vi "Destroy.vi"(8 "error in (no error)":errorcluster, 9 "force destroy? (F)":bool, 11 "State in":refnum<class "State.lvclass">) -> (0 "error out":errorcluster)   [LabVIEW 2017, in "Promise Future.lvlib" / "State.lvclass"]
uses:
  State.lvclass
  State.lvclass/State.ctl
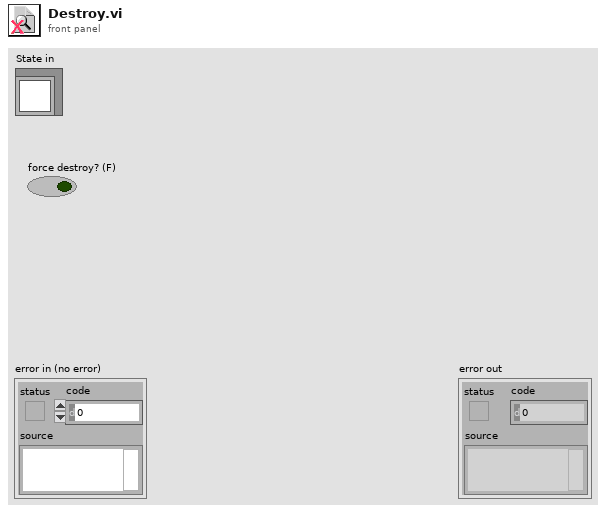
[diagram p1: front panel]
types:
  T1 = typedef "Semaphore RefNum" = refnum<k1>
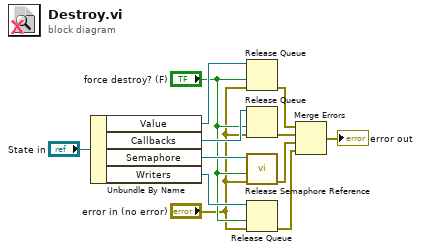
[diagram p0: block diagram]
diagram:
  n1 = Unbundle By Name("State in") -> ("Value"=w11:refnum<queue>, "Callbacks"=w9:refnum<queue>, "Semaphore"=w8:T1, "Writers"=w10:refnum<queue>)
  n2 = Release Queue(queue=w11, force destroy? (F)="force destroy? (F)", error in (no error)="error in (no error)") -> (error out=w6:errorcluster)  [unwired: 2 out]
  n3 = Release Queue(queue=w9, force destroy? (F)="force destroy? (F)", error in (no error)="error in (no error)") -> (error out=w5:errorcluster)  [unwired: 2 out]
  n4 = call <vilib>:"Release Semaphore Reference.vi"("error in (no error)"="error in (no error)", "force destroy? (F)"="force destroy? (F)", "semaphore"=w8) -> ("error out"=w4:errorcluster)  [unwired: 7 in, 1 out]
  n5 = Release Queue(queue=w10, force destroy? (F)="force destroy? (F)", error in (no error)="error in (no error)") -> (error out=w3:errorcluster)  [unwired: 2 out]
  n6 = Merge Errors(w6, w5, w4, w3) -> (→"error out":errorcluster)
